vi "Read from Network.vi"() -> ()   [LabVIEW 2015]
uses:
  <vilib>/Platform/storage/Storage.llb/usiSequenceRepresentation.ctl
  <vilib>/Platform/storage/Storage.llb/usiOverwriteOptions.ctl
  <vilib>/Platform/storage/lvStorage.llb/_openStorageWithRootAutoDetect.vi
  <vilib>/Platform/storage/lvStorage.llb/xStorage/xStorageSupp/ErrorOut.vi
  <vilib>/Platform/storage/lvStorage.llb/_createOrGetExplicitChildObject.vi
  <vilib>/Platform/storage/lvStorage.llb/_createOrGetByNameExplicitChildObject.vi
  <vilib>/Platform/storage/lvStorage.llb/__saveStringChannel.vi
  <vilib>/Platform/storage/Storage.llb/Get Object Info.vi
  <vilib>/Platform/storage/Storage.llb/__closeStorageFromObject.vi
  <vilib>/Platform/storage/lvStorage.llb/xStorage/Open Data Storage/Open Data Storage.xnode
  <vilib>/Platform/storage/lvStorage.llb/xStorage/Write Data/Write Data.xnode
  <vilib>/Platform/storage/lvStorage.llb/xStorage/Close Data Storage/Close Data Storage.xnode
panel:
  in  "stop":bool
  in  "Start":bool
  out "data out":u32[](array[numeric])
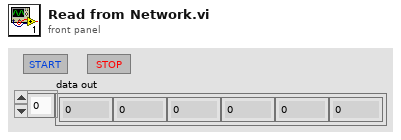
[diagram p1: front panel]
types:
  T1 = enum16{"open", "open or create", "create or replace", "create", "open (read only)"}
  T2 = enum16{"UPDATE", "READ", "QUERY", "CREATE CHILD", "CREATE", "CONNECT", "DISCONNECT"}
  T3 = typedef "usiOverwriteOptions.ctl" = enum16{"Append values", "Replace values at index", "Replace all values", "Append if timeline aligns"}
  T4 = typedef "usiSequenceRepresentation.ctl" = enum16{"explicit", "implicit"}
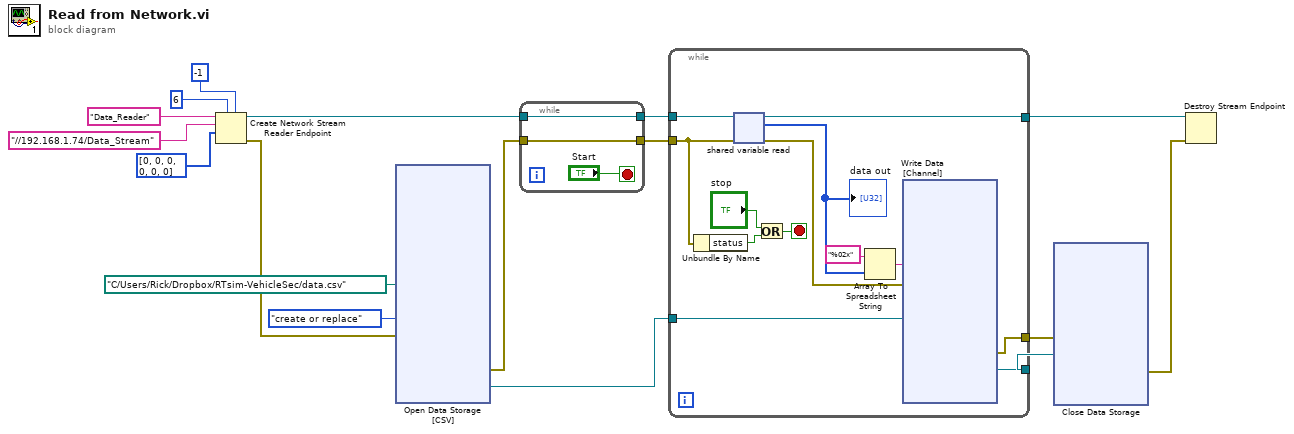
[diagram p0: block diagram]
diagram:
  n1 = Create Network Stream Reader Endpoint(5:-1 ("timeout in ms (-1)"), 7:6 ("writer buffer size"), 9:u32[] [0, 0, 0, 0, 0, 0], 10:"//192.168.1.74/Data_Stream" ("writer url"), 11:"Data_Reader" ("writer name")) -> (0:w7:errorcluster, 3:w11:refnum<k21>)  [unwired: 2 in]
  n2 = xnode "Open Data Storage\n[CSV]"("file path"=path "C:/Users/Rick/Dropbox/RTsim-VehicleSec/data.csv", "function (open:0)"=T1."create or replace", "error in (no error)"=w7) -> ("error out"=w4:errorcluster, "storage refnum (file)"=w6:refnum<k20>)  [unwired: 2 in, 1 out]
  n3 = while {
    tunnel: [w20] -> w10
    tunnel: w11 -> [w20]
    tunnel: w4 -> [w19]
    tunnel: [w19] -> w9
    stop <- "Start" stop-if-true
  }
  n4 = while {
    tunnel: [w32] -> w12
    tunnel: w10 -> [w33]
    tunnel: w9 -> [w27]
    tunnel: w6 -> [w31]
    tunnel: [w30] -> w5
    tunnel: [w28] -> w3
    stop <- w24 stop-if-true
    n5 = Unbundle By Name(w27) -> ("status"=w26:bool)
    n6 = shared-variable-read(w33, w27) -> (w32:refnum<k21>, w29:errorcluster, w23:u32[])  [unwired: 1 in, 1 out]
    "data out" <- w23
    n7 = Or(x="stop", y=w26) -> (x .or. y?=w24:bool)
    n8 = Array To Spreadsheet String(array=w23, 3:"%02x" ("format string")) -> (spreadsheet string=w22:string)  [unwired: 1 in]
    n9 = xnode "Write Data\n[Channel]"("Signal"=w22, "error in"=w29, "storage refnum (file)"=w31) -> ("error out"=w28:errorcluster, "storage refnum (file) out"=w30:refnum<k20>)  [unwired: 2 in, 1 out]
  }
  n10 = xnode "Close Data Storage\n"("error in (no error)"=w3, "storage refnum (file)"=w5) -> ("error out"=w2:errorcluster)  [unwired: 1 out]
  n11 = Destroy Stream Endpoint(8:w2, 11:w12) -> ()  [unwired: 1 out]
